vi "f_12_Eoff.vi"(0 "file path (IN)":path, 1 "Project #":string, 2 "Request #":string, 3 "TEST #":string, 5 "error in (no error)":errorcluster, 6 "VGE":dbl) -> (14 "file path (OUT)":path, 15 "Eoff (uj)":dbl, 16 "DONE Eoff":bool, 19 "error out":errorcluster)   [LabVIEW 2020]
uses:
  GlobIndSw1.vi
  <vilib>/Waveform/WDTOps.llb/WDT Waveform Duration DBL.vi
  <vilib>/Waveform/WDTOps.llb/WDT Get Waveform Subset DBL.vi
  <vilib>/measure/mamon.llb/Trigger Detection for 1 Channel.vi
  <vilib>/Analysis/NI_AALBase.lvlib
  <vilib>/measure/NI_MAPro.lvlib
panel:
  in  "Decision ?":bool
  out "Cursor a : Channel 2":dbl
  out "90% Vge":dbl
  out "Waveform Graph":waveform(dbl)[](graph)
  out "OFF Region":waveform(dbl)[](graph) caption="Eoff (uj)"
  out "Eoff Area Y-axis":dbl[](array[numeric])
  out "Eoff Area X-axis":dbl[](array[numeric])
  out "Eoff : XY Graph":cluster{"X":dbl, "Y":dbl}[](graph)
  # "Eoff: from 90% Vge to most right of whole scope screen"
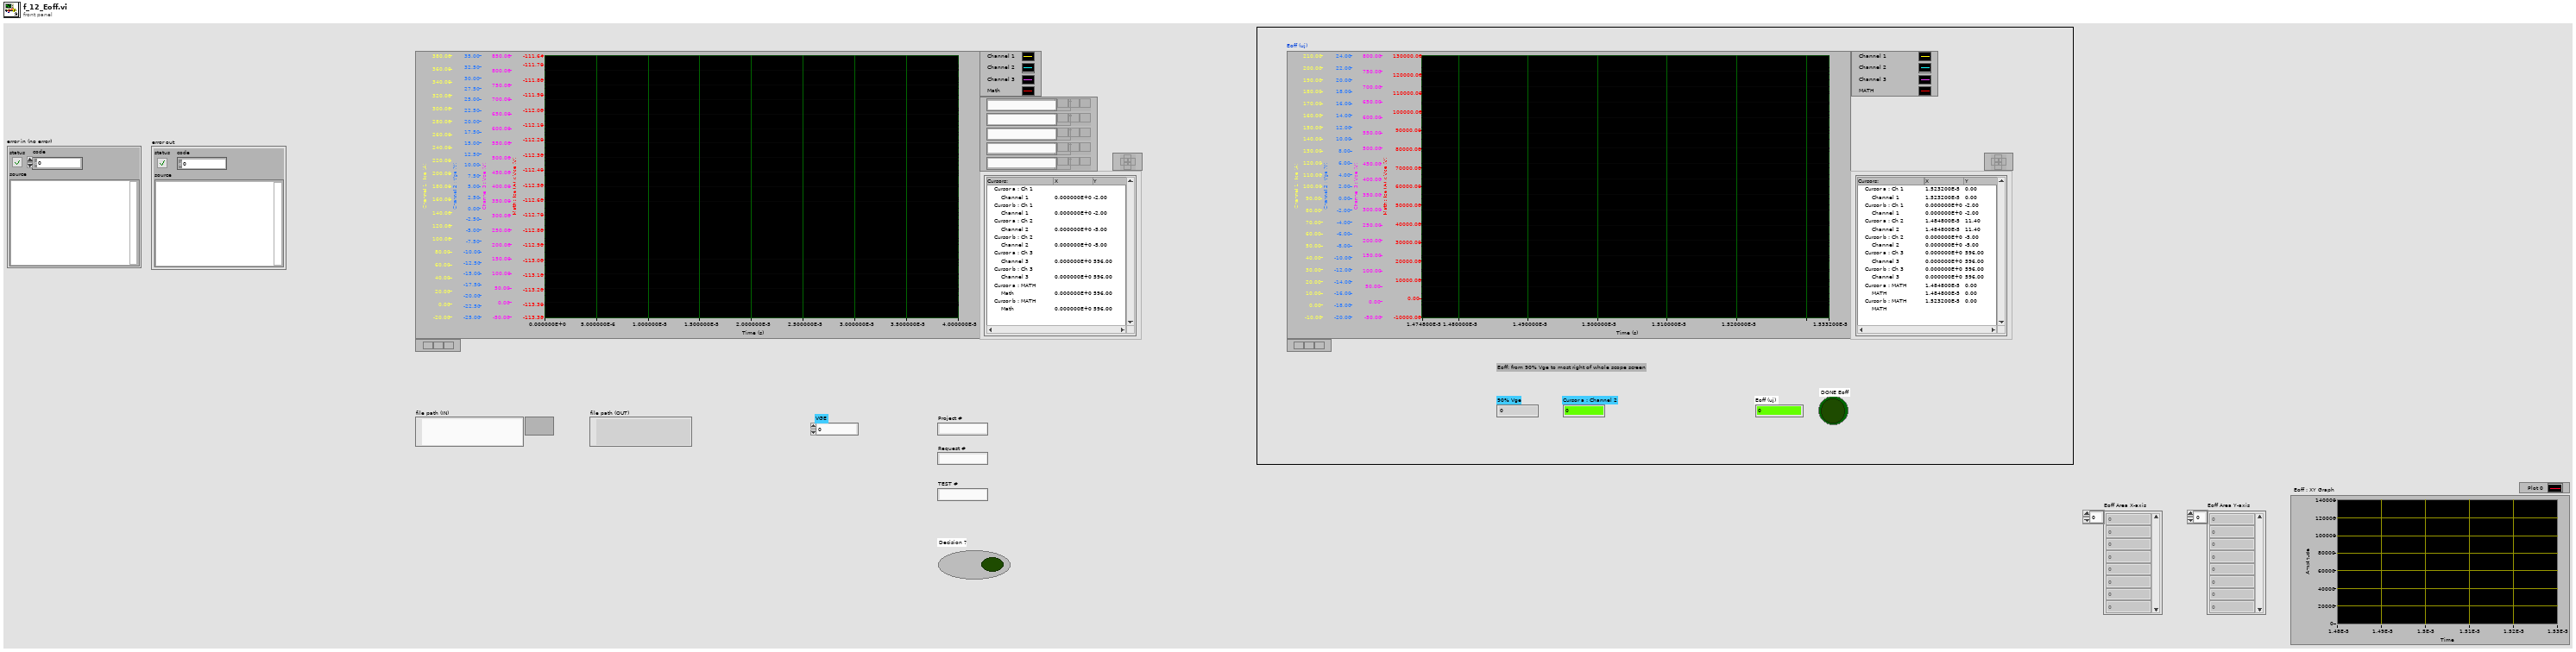
[diagram p1: front panel]
types:
  T1 = enum32{"Invalid", "Standard", "Closed", "Hidden", "Minimized", "Maximized"}
  T2 = typedef "imagedata.ctl" = cluster{"image type":i32, "image depth":i32, "image":u8[], "mask":u8[], "colors":u32[], "Rectangle":cluster{"left":i16, "top":i16, "right":i16, "bottom":i16}}
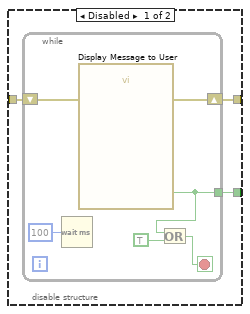
[diagram p2: hidden frame]
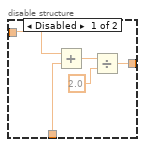
[diagram p9: hidden frame]
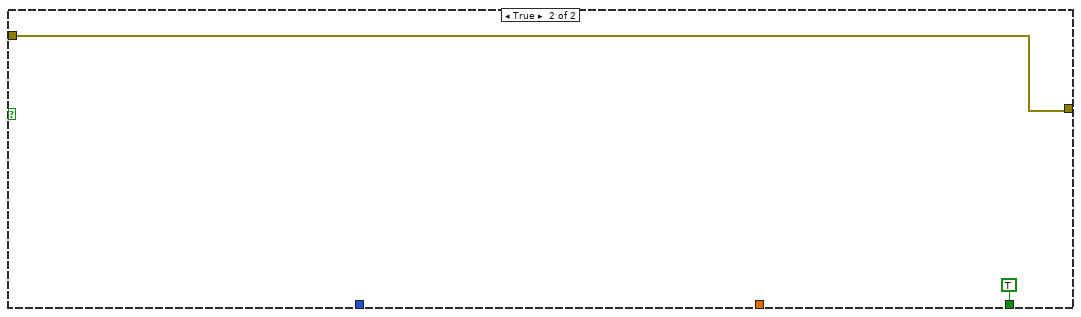
[diagram p10: hidden frame]
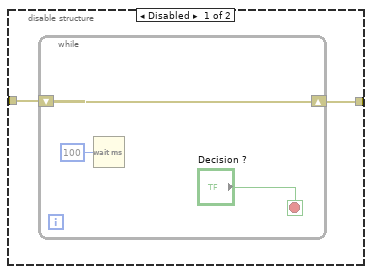
[diagram p11: hidden frame]
diagram:
  w2 = 0.0 ("Eoff (uj)")
  w6 = errorcluster {"status"=FALSE, "code"=0, "source"=""} ("error out")
  w1 = FALSE ("DONE Tdon")
  w7 = waveform(dbl)[] [] ("Waveform Graph")
  n1 = local write "error out"(w6) -> ()
  n2 = local write "error in (no error)"(w6) -> ()
  n3 = local write "DONE Eoff"(w1) -> ()
  n4 = local write "Decision ?"(w1) -> ()
  n5 = local write "Eoff (uj)"(w2) -> ()
  n6 = local write "Cursor a : Channel 2"(w2) -> ()
  n7 = local write "Waveform Graph"(w7) -> ()
  n8 = local write "OFF Region"(w7) -> ()
  n9 = flat-sequence {
    tunnel: [w15] -> w13
    tunnel: ["file path (IN)"] -> w12
    tunnel: [w25] -> w11
    tunnel: [w24] -> w10
    tunnel: w13 -> [w23]
    tunnel: w12 -> [w22]
    tunnel: w11 -> [w405]
    tunnel: [w404] -> w9
    tunnel: w10 -> [w403]
    tunnel: [w403] -> w8
    tunnel: w9 -> [w418]
    tunnel: w8 -> [w419]
    frame #0 {
      n10 = control-ref of="This VI"() -> (w17:refnum<vi>)
      n11 = invoke class="VI" method="FP.Open"(reference=w17, error in="error in (no error)", "Activate"=TRUE ("Activate?"), "State"=T1."Maximized") -> (error out=w18:errorcluster)  [unwired: 1 in, 4 out]
      n12 = property class="VI"(reference=w17, error in=w18, "Front Panel.Closeable"=TRUE ("Front Panel Window:Closeable")) -> (error out=w15:errorcluster)  [unwired: 1 out]
    }
    frame #1 {
      n13 = while {
        shift-right: [w31] -> w25
        shift-left: w23 -> [w33]
        tunnel: [w28] -> w24
        tunnel: w22 -> [w27]
        stop <- w29 stop-if-true
        n14 = flat-sequence {
          tunnel: [w74] -> w60
          tunnel: w33 -> [w80]
          tunnel: [w80] -> w32
          tunnel: w27 -> [w74]
          tunnel: w60 -> [w185]
          tunnel: [w84] -> w59
          tunnel: [w119] -> w58
          tunnel: [w109] -> w57
          tunnel: [w83] -> w56
          tunnel: [w91] -> w55
          tunnel: w32 -> [w190]
          tunnel: [w82] -> w26
          tunnel: w59 -> [w230]
          tunnel: w58 -> [w229]
          tunnel: [w242] -> w54
          tunnel: w57 -> [w241]
          tunnel: [w241] -> w53
          tunnel: [w227] -> w52
          tunnel: [w232] -> w51
          tunnel: w56 -> [w238]
          tunnel: [w238] -> w50
          tunnel: w55 -> [w231]
          tunnel: w26 -> [w226]
          tunnel: w54 -> [w272]
          tunnel: [w271] -> w49
          tunnel: w53 -> [w277]
          tunnel: [w277] -> w48
          tunnel: w52 -> [w276]
          tunnel: [w276] -> w47
          tunnel: w51 -> [w275]
          tunnel: [w275] -> w46
          tunnel: w50 -> [w274]
          tunnel: [w274] -> w45
          tunnel: w49 -> [w289]
          tunnel: [w280] -> w44
          tunnel: w48 -> [w290]
          tunnel: [w290] -> w43
          tunnel: w47 -> [w288]
          tunnel: [w288] -> w42
          tunnel: w46 -> [w287]
          tunnel: [w287] -> w41
          tunnel: w45 -> [w285]
          tunnel: w44 -> [w372]
          tunnel: [w371] -> w40
          tunnel: w43 -> [w379]
          tunnel: [w379] -> w39
          tunnel: w42 -> [w368]
          tunnel: w41 -> [w367]
          tunnel: [w367] -> w38
          tunnel: [w368] -> w37
          tunnel: w40 -> [w390]
          tunnel: [w391] -> w36
          tunnel: w39 -> [w392]
          tunnel: [w392] -> w35
          tunnel: w38 -> [w385]
          tunnel: w37 -> [w384]
          tunnel: w36 -> [w395]
          tunnel: w35 -> [w393]
          tunnel: [w394] -> w34
          tunnel: [w393] -> w28
          frame #0 {
            w73 = FALSE ("DONE Tdon")
            w79 = waveform(dbl)[] [] ("Waveform Graph")
            w78 = 0.0 ("Eoff (uj)")
            n15 = local write "DONE Eoff"(w73) -> ()
            n16 = local write "Decision ?"(w73) -> ()
            n17 = local write "Eoff (uj)"(w78) -> ()
            n18 = local write "Cursor a : Channel 2"(w78) -> ()
            n19 = Wait (ms)(milliseconds to wait=u32 400) -> ()  [unwired: 1 out]
            n20 = local write "Waveform Graph"(w79) -> ()
            n21 = local write "OFF Region"(w79) -> ()
            n22 = local write "Eoff Area Y-axis"(dbl[] [] ("Eoff Area X-axis")) -> ()
            n23 = local write "Eoff Area X-axis"(dbl[] [] ("Eoff Area Y-axis")) -> ()
            n24 = local write "Eoff : XY Graph"(cluster{"X":dbl, "Y":dbl}[] [] ("Eoff : XY Graph")) -> ()
          }
          frame #1 {
            w85 = 0.0 ("start samples/time")
            w98 = u16 1 items=["Samples", "Relative Time"] ("start/duration format")
            w167 = u16 1 items=["Samples", "Relative Time"] ("start/duration format")
            w177 = u16 1 items=["Samples", "Relative Time"] ("start/duration format")
            w178 = u16 1 items=["Samples", "Relative Time"] ("start/duration format")
            # "Channel 3"
            # "Channel 1"
            # "Channel MATH"
            # "MATH = Ch1 x Ch3"
            # "Channel 1"
            # "Channel 3"
            # "Channel 2"
            # "dt"
            # "Ch2"
            # "Ch1"
            n25 = call "3_ReadDatatoWaveform.vi"("error in (no error)"=w190, "file path (IN)"=w185) -> ("error out"=w86:errorcluster, "Waveform Graph"=→"Waveform Graph":waveform(dbl)[], "file path (OUT)"=w109:path, "dt"=w186:dbl, "Ch 2 Data"=w183:dbl[], "Ch 3 Data"=w187:dbl[], "Ch 1 Data"=w184:dbl[])  [unwired: 3 in]
            n26 = Wait (ms)(milliseconds to wait=u32 400) -> ()  [unwired: 1 out]
            n27 = call <vilib>:"Beep.vi"("use system alert? (T)"=FALSE, "duration (msec)"=u32 200, "frequency (Hz)"=u32 2000) -> ()  [unwired: 9 in]
            n28 = To Time Stamp(1:0.0 ("number")) -> (0:w188:timestamp)
            n29 = disable-structure shown="Enabled" {
              disable-tunnel: w188 -> [w221 _]
              disable-tunnel: w186 -> [w220 _]
              disable-tunnel: w187 -> [w219 _]
              disable-tunnel: [w218 _] -> w105
              frame Enabled {
                # "Channel 3"
                n30 = Bundle By Name("Y"=w219, "dt"=w220, "t0"=w221) -> (w218:waveform(dbl))  [unwired: 1 in]
              }
              frame Disabled {
              }
            }
            n31 = disable-structure shown="Enabled" {
              disable-tunnel: w188 -> [w217 _]
              disable-tunnel: w186 -> [w216 _]
              disable-tunnel: w183 -> [w215 _]
              disable-tunnel: [w214 _] -> w87
              frame Enabled {
                # "Channel 2"
                n32 = Bundle By Name("Y"=w215, "dt"=w216, "t0"=w217) -> (w214:waveform(dbl))  [unwired: 1 in]
              }
              frame Disabled {
              }
            }
            n33 = disable-structure shown="Enabled" {
              disable-tunnel: w188 -> [w213 _]
              disable-tunnel: w186 -> [w212 _]
              disable-tunnel: w184 -> [w211 _]
              disable-tunnel: [w210 _] -> w106
              frame Enabled {
                # "Channel 1"
                n34 = Bundle By Name("Y"=w211, "dt"=w212, "t0"=w213) -> (w210:waveform(dbl))  [unwired: 1 in]
              }
              frame Disabled {
              }
            }
            n35 = Unbundle By Name(w105) -> ("Y"=w102:dbl[])
            n36 = Unbundle By Name(w106) -> ("Y"=w103:dbl[], "dt"=w92:dbl, "t0"=w104:timestamp)
            n37 = disable-structure shown="Enabled" {
              disable-tunnel: w87 -> [w203 _]
              disable-tunnel: w86 -> [w195 _]
              disable-tunnel: [w194 _] -> w88
              disable-tunnel: [w193 _] -> w84
              disable-tunnel: w85 -> [w192 _]
              frame Enabled {
                w197 = u16 1 items=["Samples", "Relative Time"] ("start/duration format")
                # "Channel 2 - Filtered"
                # "Median"
                n38 = global read "GlobIndSw1.vi" "Median Filter Rank"() -> (w191:i32)
                n39 = Unbundle By Name(w203) -> ("Y"=w206:dbl[], "dt"=w204:dbl)
                n40 = call <vilib>:"Median Filter.vi"("right rank"=w191, "left rank"=w191, "X"=w206) -> ("Filtered X"=w205:dbl[])  [unwired: 7 in, 1 out]
                n41 = Bundle By Name("Y"=w205, "dt"=w204) -> (w196:waveform(dbl))  [unwired: 1 in]
                n42 = call-poly <vilib>:"Waveform Duration.vi"("error in (no error)"=w195, "waveform in"=w196) -> ("error out"=w200:errorcluster, "duration"=w202:dbl, "waveform out"=w201:waveform(dbl))  [unwired: 7 in]
                n43 = Divide(x=w202, y=2.0) -> (x/y=w199:dbl)
                n44 = call-poly <vilib>:"Get Waveform Subset.vi"("start/duration format"=w197, "error in (no error)"=w200, "duration"=w199, "start samples/time"=w192, "waveform in"=w201) -> ("error out"=w194:errorcluster, "waveform out"=w193:waveform(dbl))  [unwired: 1 in, 2 out]
              }
              frame Disabled {
              }
            }
            n45 = for {
              tunnel: w103 -> [w209] mode=indexing
              tunnel: w102 -> [w208] mode=indexing
              tunnel: [w207] -> w101 mode=indexing
              n46 = Multiply(x=w209, y=w208) -> (x*y=w207:dbl)
            }
            n47 = Bundle By Name("Y"=w101, "dt"=w92, "t0"=w104) -> (w93:waveform(dbl))  [unwired: 1 in]
            n48 = call-poly <vilib>:"Waveform Duration.vi"("error in (no error)"=w86, "waveform in"=w93) -> ("error out"=w94:errorcluster, "duration"=w96:dbl, "waveform out"=w99:waveform(dbl))  [unwired: 7 in]
            n49 = call-poly <vilib>:"Waveform Duration.vi"("error in (no error)"=w86, "waveform in"=w105) -> ("error out"=w171:errorcluster, "duration"=w169:dbl, "waveform out"=w107:waveform(dbl))  [unwired: 7 in]
            n50 = call-poly <vilib>:"Waveform Duration.vi"("error in (no error)"=w86, "waveform in"=w87) -> ("error out"=w172:errorcluster, "duration"=w175:dbl, "waveform out"=w173:waveform(dbl))  [unwired: 7 in]
            n51 = call-poly <vilib>:"Waveform Duration.vi"("error in (no error)"=w86, "waveform in"=w106) -> ("error out"=w182:errorcluster, "duration"=w179:dbl, "waveform out"=w181:waveform(dbl))  [unwired: 7 in]
            n52 = Divide(x=w96, y=2.0) -> (x/y=w97:dbl)
            n53 = Divide(x=w169, y=2.0) -> (x/y=w168:dbl)
            n54 = Divide(x=w175, y=2.0) -> (x/y=w176:dbl)
            n55 = Divide(x=w179, y=2.0) -> (x/y=w91:dbl)
            n56 = call-poly <vilib>:"Get Waveform Subset.vi"("start/duration format"=w177, "error in (no error)"=w172, "duration"=w176, "start samples/time"=w85, "waveform in"=w173) -> ("error out"=w164:errorcluster, "waveform out"=w120:waveform(dbl))  [unwired: 1 in, 2 out]
            n57 = call-poly <vilib>:"Get Waveform Subset.vi"("start/duration format"=w167, "error in (no error)"=w171, "duration"=w168, "start samples/time"=w85, "waveform in"=w107) -> ("error out"=w90:errorcluster, "waveform out"=w108:waveform(dbl))  [unwired: 1 in, 2 out]
            n58 = call-poly <vilib>:"Get Waveform Subset.vi"("start/duration format"=w178, "error in (no error)"=w182, "duration"=w91, "start samples/time"=w85, "waveform in"=w181) -> ("error out"=w165:errorcluster, "waveform out"=w82:waveform(dbl))  [unwired: 1 in, 2 out]
            n59 = call-poly <vilib>:"Get Waveform Subset.vi"("start/duration format"=w98, "error in (no error)"=w94, "duration"=w97, "start samples/time"=w85, "waveform in"=w99) -> ("error out"=w89:errorcluster, "waveform out"=w83:waveform(dbl))  [unwired: 1 in, 2 out]
            n60 = Build Array(w82, w120, w108, w83) -> (→"OFF Region":waveform(dbl)[])
            n61 = Merge Errors(w165, w164, w90, w89, w88) -> (w117:errorcluster)
            n62 = property on="OFF Region" class="WFGraph (strict)"(error in=w117) -> (error out=w116:errorcluster, "Width"=w115:u32)  [unwired: 1 in, 1 out]
            n63 = property on="OFF Region" class="WFGraph (strict)"(error in=w116, "Caption.Justify"=enum16{"Left", "Center", "Right"}."Left" ("Caption.Justification"), "Caption.Width"=w115, "Caption.FontBold"=TRUE ("Caption.Font:Bold"), "Caption.FontColor"=u32 16860 ("Caption.Font:Color"), "Caption.FontSize"=u32 24 ("Caption.Font:Size"), "Caption.Text"="Eoff (uj)") -> (error out=w111:errorcluster)  [unwired: 1 in, 1 out]
            n64 = property on="OFF Region" class="WFGraph (strict)"(error in=w111, "XScale.Offset"=w85) -> (error out=w144:errorcluster)  [unwired: 1 in, 1 out]
            n65 = property on="OFF Region" class="WFGraph (strict)"(error in=w144, "Active Cursor"=u32 0, "Cursor.Cursor X"=0.0 ("Cursor.Cursor Position:Cursor X"), "Cursor.Cursor Y"=0.0 ("Cursor.Cursor Position:Cursor Y"), "Cursor.Visible"=FALSE) -> (error out=w143:errorcluster)  [unwired: 1 in, 1 out]
            n66 = property on="OFF Region" class="WFGraph (strict)"(error in=w143, "Active Cursor"=u32 1, "Cursor.Cursor X"=0.0 ("Cursor.Cursor Position:Cursor X"), "Cursor.Cursor Y"=0.0 ("Cursor.Cursor Position:Cursor Y"), "Cursor.Visible"=FALSE) -> (error out=w142:errorcluster)  [unwired: 1 in, 1 out]
            n67 = property on="OFF Region" class="WFGraph (strict)"(error in=w142, "Active Cursor"=u32 2, "Cursor.Cursor X"=0.0 ("Cursor.Cursor Position:Cursor X"), "Cursor.Cursor Y"=0.0 ("Cursor.Cursor Position:Cursor Y"), "Cursor.Visible"=FALSE) -> (error out=w141:errorcluster)  [unwired: 1 in, 1 out]
            n68 = property on="OFF Region" class="WFGraph (strict)"(error in=w141, "Active Cursor"=u32 3, "Cursor.Cursor X"=0.0 ("Cursor.Cursor Position:Cursor X"), "Cursor.Cursor Y"=0.0 ("Cursor.Cursor Position:Cursor Y"), "Cursor.Visible"=FALSE) -> (error out=w124:errorcluster)  [unwired: 1 in, 1 out]
            n69 = property on="OFF Region" class="WFGraph (strict)"(error in=w124, "Active Cursor"=u32 4, "Cursor.Cursor X"=0.0 ("Cursor.Cursor Position:Cursor X"), "Cursor.Cursor Y"=0.0 ("Cursor.Cursor Position:Cursor Y"), "Cursor.Visible"=FALSE) -> (error out=w123:errorcluster)  [unwired: 1 in, 1 out]
            n70 = property on="OFF Region" class="WFGraph (strict)"(error in=w123, "Active Cursor"=u32 5, "Cursor.Cursor X"=0.0 ("Cursor.Cursor Position:Cursor X"), "Cursor.Cursor Y"=0.0 ("Cursor.Cursor Position:Cursor Y"), "Cursor.Visible"=FALSE) -> (error out=w122:errorcluster)  [unwired: 1 in, 1 out]
            n71 = property on="OFF Region" class="WFGraph (strict)"(error in=w122, "Active Cursor"=u32 6, "Cursor.Cursor X"=0.0 ("Cursor.Cursor Position:Cursor X"), "Cursor.Cursor Y"=0.0 ("Cursor.Cursor Position:Cursor Y"), "Cursor.Visible"=FALSE) -> (error out=w121:errorcluster)  [unwired: 1 in, 1 out]
            n72 = property on="OFF Region" class="WFGraph (strict)"(error in=w121, "Active Cursor"=u32 7, "Cursor.Cursor X"=0.0 ("Cursor.Cursor Position:Cursor X"), "Cursor.Cursor Y"=0.0 ("Cursor.Cursor Position:Cursor Y"), "Cursor.Visible"=FALSE) -> (error out=w119:errorcluster)  [unwired: 1 in, 1 out]
          }
          frame #2 {
            w236 = u16 0 items=["Falling Edge", "Rising Edge"] ("trigger slope")
            w237 = u16 1 items=["Index", "Time"] ("location mode")
            # "Cursor a : Channel 1"
            # "Channel 1"
            # "Cursor a : Channel 2"
            # "End Time 1st Cursor"
            # "2nd PARAMETER"
            # "MOST RIGHT SCREEN"
            # "1st PARAMETER"
            # "Channel 2"
            n73 = Wait (ms)(milliseconds to wait=u32 500) -> ()  [unwired: 1 out]
            n74 = call <vilib>:"Beep.vi"("use system alert? (T)"=FALSE, "duration (msec)"=u32 200, "frequency (Hz)"=u32 2000) -> ()  [unwired: 9 in]
            n75 = Divide(x=90.0, y=100.0) -> (x/y=w255:dbl)
            n76 = Multiply(x=w255, y="VGE") -> (x*y=w234:dbl)
            "90% Vge" <- w234
            n77 = Add(x=w234, y=0.2) -> (x+y=w225:dbl)
            n78 = Divide(x=w225, y=10.0) -> (x/y=w223:dbl)
            n79 = call-poly <vilib>:"Basic Level Trigger Detection.vi"("signal in"=w230, "level"=w225, "hysteresis"=w223, "location mode"=w237, "error in (no error)"=w229, "trigger slope"=w236) -> ("trigger location"=w232:dbl, "error out"=w233:errorcluster)  [unwired: 7 in, 1 out]
            n80 = disable-structure shown="Enabled" {
              disable-tunnel: [w261 _] -> w228
              disable-tunnel: w229 -> [w260 _]
              disable-tunnel: w226 -> [w259 _]
              disable-tunnel: [w257 _] -> w227
              frame Enabled {
                w263 = u16 0 items=["Falling Edge", "Rising Edge"] ("trigger slope")
                w262 = u16 1 items=["Index", "Time"] ("location mode")
                n81 = call-poly <vilib>:"Basic Level Trigger Detection.vi"("signal in"=w259, "level"=0.2, "hysteresis"=10.0, "location mode"=w262, "error in (no error)"=w260, "trigger slope"=w263) -> ("trigger location"=w257:dbl, "error out"=w261:errorcluster)  [unwired: 7 in, 1 out]
              }
              frame Disabled {
              }
            }
            n82 = disable-structure shown="Enabled" {
              disable-tunnel: w232 -> [w266 _]
              disable-tunnel: w231 -> [w265 _]
              disable-tunnel: [w264 _] -> _
              frame Disabled {
                n83 = Add(x=w265, y=w266) -> (x+y=w268:dbl)
                n84 = Divide(x=w268, y=2.0) -> (x/y=w264:dbl)
              }
              frame Enabled {
              }
            }
            n85 = disable-structure shown="Disabled" {
              frame Disabled {
                # "3"
                # "Cursor b : Channel 2"
              }
              frame Enabled {
              }
            }
            n86 = property on="OFF Region" class="WFGraph (strict)"(error in=w233, "Active Cursor"=u32 2, "Cursor.Cursor X"=w232, "Cursor.Visible"=TRUE, "Cursor.Cursor Name Visible"=TRUE) -> (error out=w243:errorcluster)  [unwired: 1 in, 1 out]
            n87 = property on="OFF Region" class="WFGraph (strict)"(error in=w228, "Active Cursor"=u32 0, "Cursor.Cursor X"=w227, "Cursor.Visible"=TRUE, "Cursor.Cursor Name Visible"=TRUE) -> (error out=w244:errorcluster)  [unwired: 1 in, 1 out]
            n88 = Merge Errors(w244, w243) -> (w242:errorcluster)
          }
          frame #3 {
            # "Cursor a : Channel 2"
            n89 = property on="OFF Region" class="WFGraph (strict)"(error in=w272, "Active Cursor"=u32 2) -> (error out=w271:errorcluster, "Cursor.Cursor Y"=→"Cursor a : Channel 2":dbl)  [unwired: 1 in, 1 out]
            n90 = Wait (ms)(milliseconds to wait=u32 300) -> ()  [unwired: 1 out]
          }
          frame #4 {
            n91 = flat-sequence {
              tunnel: w289 -> [w294]
              tunnel: w288 -> [w296]
              tunnel: w287 -> [w295]
              tunnel: [w291] -> w286
              tunnel: w286 -> [w305]
              tunnel: w284 -> [w304]
              tunnel: [w303] -> w283
              tunnel: w283 -> [w346]
              tunnel: [w348] -> w282
              tunnel: [w347] -> w281
              tunnel: [w346] -> w279
              tunnel: w282 -> [w354]
              tunnel: w281 -> [w353]
              tunnel: [w352] -> w280
              tunnel: w279 -> [w352]
              frame #0 {
                # "Cursor a : MATH"
                # "Cursor b : MATH"
                n92 = property on="OFF Region" class="WFGraph (strict)"(error in=w294, "Active Cursor"=u32 7, "Cursor.Cursor X"=w296, "Cursor.Visible"=TRUE, "Cursor.Cursor Name Visible"=TRUE) -> (error out=w292:errorcluster)  [unwired: 1 in, 1 out]
                n93 = property on="OFF Region" class="WFGraph (strict)"(error in=w294, "Active Cursor"=u32 6, "Cursor.Cursor X"=w295, "Cursor.Visible"=TRUE, "Cursor.Cursor Name Visible"=TRUE) -> (error out=w293:errorcluster)  [unwired: 1 in, 1 out]
                n94 = Merge Errors(w292, w293) -> (w291:errorcluster)
              }
              frame #1 {
                n95 = while {
                  tunnel: w305 -> [w313]
                  tunnel: w304 -> [w307]
                  tunnel: [w306] -> w303
                  i -> [w308]
                  stop <- w311 stop-if-true
                  # "Cursor b : MATH"
                  # "Cursor a : MATH"
                  n96 = property on="OFF Region" class="WFGraph (strict)"(error in=w313, "Active Cursor"=u32 7) -> (error out=w317:errorcluster, "Cursor.Cursor X"=w319:dbl)  [unwired: 1 in, 1 out]
                  n97 = property on="OFF Region" class="WFGraph (strict)"(error in=w313, "Active Cursor"=u32 6) -> (error out=w316:errorcluster, "Cursor.Cursor X"=w318:dbl)  [unwired: 1 in, 1 out]
                  n98 = Merge Errors(w316, w317) -> (w309:errorcluster)
                  n99 = Equal?(x=w318, y=w319) -> (x = y?=w312:bool)
                  n100 = case shown="False" w312 {
                    tunnel: [FALSE TRUE] -> w311
                    tunnel: w309 -> [w324 w344]
                    tunnel: w308 -> [w323 _]
                    tunnel: w307 -> [w321 _]
                    tunnel: [w320 w344] -> w306
                    frame False {
                      n101 = flat-sequence {
                        tunnel: w324 -> [w334]
                        tunnel: w323 -> [w329]
                        tunnel: [w326] -> w322
                        tunnel: w322 -> [w339]
                        tunnel: w321 -> [w337]
                        tunnel: [w336] -> w320
                        frame #0 {
                          # "Cursor a : MATH"
                          n102 = property on="OFF Region" class="WFGraph (strict)"(error in=w334, "Active Cursor"=u32 6) -> (error out=w326:errorcluster, "Cursor.Cursor X"=w331:dbl, "Cursor.Cursor Y"=w330:dbl)  [unwired: 1 in, 1 out]
                          n103 = local read "Eoff Area Y-axis"() -> (w332:dbl[])
                          n104 = local read "Eoff Area X-axis"() -> (w333:dbl[])
                          n105 = Insert Into Array(array=w332, index=w329, new element=w330) -> (w327:dbl[])
                          n106 = Insert Into Array(array=w333, index=w329, new element=w331) -> (w328:dbl[])
                          n107 = local write "Eoff Area X-axis"(w328) -> ()
                          n108 = local write "Eoff Area Y-axis"(w327) -> ()
                        }
                        frame #1 {
                          # "Cursor a : MATH"
                          # "Cursor a : MATH"
                          n109 = property on="OFF Region" class="WFGraph (strict)"(error in=w339, "Active Cursor"=u32 6) -> (error out=w338:errorcluster, "Cursor.Cursor X"=w341:dbl)  [unwired: 1 in, 1 out]
                          n110 = Add(x=w341, y=w337) -> (x+y=w340:dbl)
                          n111 = property on="OFF Region" class="WFGraph (strict)"(error in=w338, "Active Cursor"=u32 6, "Cursor.Cursor X"=w340) -> (error out=w336:errorcluster)  [unwired: 1 in, 1 out]
                        }
                      }
                    }
                    frame True {
                    }
                  }
                  n112 = Wait (ms)(milliseconds to wait=u32 1) -> ()  [unwired: 1 out]
                }
              }
              frame #2 {
                n113 = local read "Eoff Area X-axis"() -> (w348:dbl[])
                n114 = local read "Eoff Area Y-axis"() -> (w347:dbl[])
                n115 = Build Cluster Array(w348, w347) -> (w349:cluster{dbl, dbl}[])
                n116 = local write "Eoff : XY Graph"(w349) -> ()
                n117 = Wait (ms)(milliseconds to wait=u32 50) -> ()  [unwired: 1 out]
              }
              frame #3 {
                n118 = Wait (ms)(milliseconds to wait=u32 50) -> ()  [unwired: 1 out]
                n119 = Delete From Array(array=w354, index=0) -> (array with subset deleted=w364:dbl[])  [unwired: 1 in, 1 out]
                n120 = Delete From Array(array=w353, index=0) -> (array with subset deleted=w358:dbl[])  [unwired: 1 in, 1 out]
                n121 = Subtract(x=w364, y=w354) -> (x-y=w363:dbl[])
                n122 = Add(x=w358, y=w353) -> (x+y=w362:dbl[])
                n123 = Compound Arithmetic op=MULTIPLY(w363, w362, invert 2.0 ("Numeric")) -> (w360:dbl[])
                n124 = Add Array Elements(numeric array=w360) -> (sum=w356:dbl)
                n125 = Multiply(x=w356, y=1000000.0) -> (x*y=→"Eoff (uj)":dbl)
              }
            }
            n126 = Unbundle By Name(w285) -> ("dt"=w284:dbl)
            n127 = Wait (ms)(milliseconds to wait=u32 300) -> ()  [unwired: 1 out]
          }
          frame #5 {
            # "Cursor a : MATH"
            # "Cursor b : MATH"
            n128 = property on="OFF Region" class="WFGraph (strict)"(error in=w372, "Active Cursor"=u32 7, "Cursor.Cursor X"=w368, "Cursor.Visible"=TRUE, "Cursor.Cursor Name Visible"=TRUE) -> (error out=w369:errorcluster)  [unwired: 1 in, 1 out]
            n129 = property on="OFF Region" class="WFGraph (strict)"(error in=w372, "Active Cursor"=u32 6, "Cursor.Cursor X"=w367, "Cursor.Visible"=TRUE, "Cursor.Cursor Name Visible"=TRUE) -> (error out=w370:errorcluster)  [unwired: 1 in, 1 out]
            n130 = Wait (ms)(milliseconds to wait=u32 300) -> ()  [unwired: 1 out]
            n131 = Merge Errors(w369, w370) -> (w371:errorcluster)
          }
          frame #6 {
            # "2nd Cursor"
            # "1st Cursor"
            n132 = Subtract(x=w385, y=1e-07) -> (x-y=w386:dbl)
            n133 = Add(x=w384, y=1e-07) -> (x+y=w387:dbl)
            n134 = property on="OFF Region" class="WFGraph (strict)"(error in=w390, "XScale.Minimum"=w386, "XScale.Maximum"=w387) -> (error out=w391:errorcluster)  [unwired: 1 in, 1 out]
            n135 = Wait (ms)(milliseconds to wait=u32 300) -> ()  [unwired: 1 out]
            n136 = call <vilib>:"Beep.vi"("use system alert? (T)"=FALSE, "duration (msec)"=u32 200, "frequency (Hz)"=u32 2000) -> ()  [unwired: 9 in]
          }
          frame #7 {
            n137 = disable-structure shown="Enabled" {
              disable-tunnel: w395 -> [w397 w401]
              disable-tunnel: [w396 w401] -> w394
              frame Disabled {
                n138 = while {
                  shift-right: [w398] -> w396
                  shift-left: w397 -> [w398]
                  stop <- "Decision ?" stop-if-true
                  n139 = Wait (ms)(milliseconds to wait=u32 100) -> ()  [unwired: 1 out]
                }
              }
              frame Enabled {
              }
            }
          }
        }
        n140 = disable-structure shown="Enabled" {
          disable-tunnel: w34 -> [w63 w71]
          disable-tunnel: [w62 w71] -> w31
          disable-tunnel: [w61 TRUE ("NO")] -> w29
          frame Disabled {
            n141 = while {
              tunnel: [w65] -> w61
              shift-right: [w68] -> w62
              shift-left: w63 -> [w69]
              stop <- w67 stop-if-true
              n142 = Wait (ms)(milliseconds to wait=u32 100) -> ()  [unwired: 1 out]
              n143 = call "Display Message to User"("error in (no error)"=w69) -> ("error out"=w68:errorcluster, "NO"=w65:bool)  [unwired: 9 in]
              n144 = Or(x=w65, y=TRUE) -> (x .or. y?=w67:bool)
            }
          }
          frame Enabled {
          }
        }
        n145 = Wait (ms)(milliseconds to wait=u32 100) -> ()  [unwired: 1 out]
      }
    }
    frame #2 {
      w409 = "_"
      n146 = Wait (ms)(milliseconds to wait=u32 300) -> ()  [unwired: 1 out]
      n147 = invoke on="OFF Region" class="WFGraph (strict)" method="Get Image"(error in=w405) -> (error out=w411:errorcluster, "image data"=w414:T2)  [unwired: 5 in, 4 out]
      n148 = Concatenate Strings("C:\\Inductive_Switching_Project\\IndSw_Image\\" ("string"), "Project #", w409, "Request #", w409, "TEST #", w409, "Eoff" ("string"), ".png" ("string")) -> (w415:string)
      n149 = String To Path(string=w415) -> (path=w413:path)
      n150 = call <vilib>:"Write PNG File.vi"("error in (no error)"=w411, "image data"=w414, "path to PNG file"=w413) -> ("error out"=w404:errorcluster)  [unwired: 7 in, 1 out]
      "DONE Eoff" <- TRUE ("DONE Tdon")
    }
    frame #3 {
      n151 = disable-structure shown="Enabled" {
        disable-tunnel: w418 -> [w420 _]
        frame Enabled {
          n152 = control-ref of="This VI"() -> (w421:refnum<vi>)
          n153 = invoke class="VI" method="FP.Close"(reference=w421, error in=w420) -> ()  [unwired: 1 in, 3 out]
        }
        frame Disabled {
        }
      }
      "error out" <- w418
      "file path (OUT)" <- w419
    }
  }
  "Eoff : XY Graph" <- cluster{"X":dbl, "Y":dbl}[] [] ("Eoff : XY Graph")
  "Eoff Area X-axis" <- dbl[] [] ("Eoff Area X-axis")
  "Eoff Area Y-axis" <- dbl[] [] ("Eoff Area Y-axis")
